vi "Mutate.RemoveOldInsertionPaletteItemsProject.vi"() -> ()   [LabVIEW 2013, in "VeriStand Steps Version Mutation.lvlib"]
uses:
  VeriStand Steps Version Mutation.lvlib
  <vilib>/xml/Load XML File.vi
  <vilib>/xml/Close Reference(Node).vi
  <vilib>/xml/Close Reference(NNMap).vi
  <vilib>/ni/Simple XML/_polymorphics/Create Tag - Child with Text.vi
  <vilib>/xml/NI_XML.lvlib
  <resource>/objmgr/DOMUserDefRef.rc
  <vilib>/ni/Simple XML/Simple XML.lvlib
panel:
  out "New Assembly Reference Include Strings":string[](array[string])=["NationalInstruments.TestStand.Interop.API, Version=1.2.3.4, Culture=neutral, PublicKeyToken=ad9244eb3b825cd8, processorArchitecture=MSIL", "NationalInstruments.TestStand.Interop.UI.AxControls, Version=1.2.3.4, Culture=neutral, PublicKeyToken=ad9244eb3b825cd8, processorArchitecture=MSIL", "NationalInstruments.TestStand.Interop.Utility, Version=5.6.7.8, Culture=neutral, processorArchitecture=x86"]
  out "New Assembly HintPath Properties":string[](array[string])=["..\\..\\..\\..\\..\\..\\..\\..\\..\\Program Files (x86)\\National Instruments\\TestStand 2013\\API\\DotNet\\Assemblies\\CurrentVersion\\NationalInstruments.TestStand.Interop.API.dll", "..\\..\\..\\..\\..\\..\\..\\..\\..\\Program Files (x86)\\National Instruments\\TestStand 2013\\API\\DotNet\\Assemblies\\CurrentVersion\\NationalInstruments.TestStand.Interop.UI.AxControls.dll", "..\\..\\..\\..\\..\\..\\..\\..\\..\\Program Files (x86)\\National Instruments\\TestStand 2013\\Bin\\NationalInstruments.TestStand.Utility.dll"]
  in  "New TS Version":dbl=2013.0 format="%#_6f"
  out "error out":errorcluster={"status"=TRUE, "code"=-2628, "source"="Invoke Node in NI_XML.lvlib:Load XML File.vi->Assembly Redirection VIs.lvlib:Redirect Assemblies in RemoveOldInsertionPaletteItems Project XML.vi"}
  in  "Path to New XML File":path=path "C:/Users/achurch/Documents/Source/XML Assembly Redirection Project/Examples XML Files/RemoveOldInsertionPaletteItems_mod.csproj" caption="Path to New RemoveOldInsertionPaletteItems project file"
  in  "New TS Utility Assembly Version":string="5.6.7.8"
  in  "New TS Interop Assembly Version":string="1.2.3.4"
  in  "XML file path":path=path "C:/Users/achurch/Documents/Source/XML Assembly Redirection Project/Examples XML Files/RemoveOldInsertionPaletteItems.csproj" caption="Path to Old RemoveOldInsertionPaletteItems project file"
  # "Arguments\n1: Old Project Path\n2: New Project Path\n3: New TS Version (2014)\n4: New TS Utility Version (2014.0.0.0)\n5: New TS Interop Version (2014.0.0.0)"
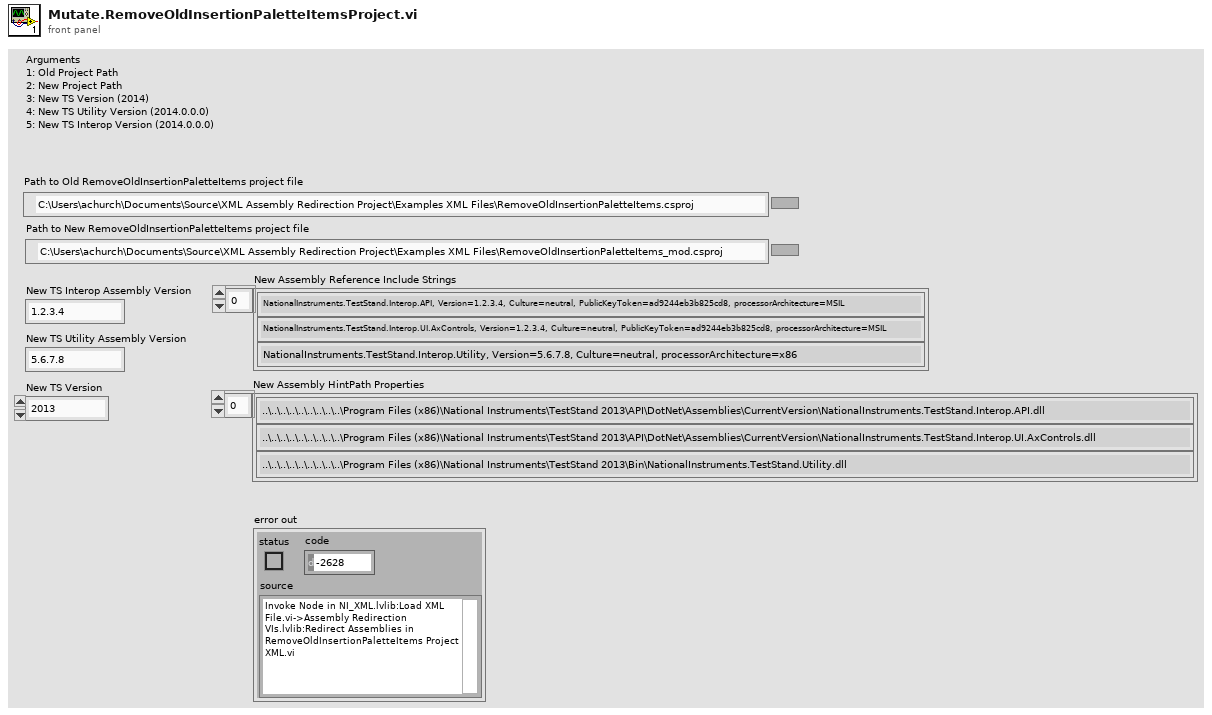
[diagram p1: front panel]
types:
  T1 = enum32{"invalid app kind", "Development System", "Run Time System", "Student Edition", "Embedded LabVIEW", "Evaluation", "Custom"}
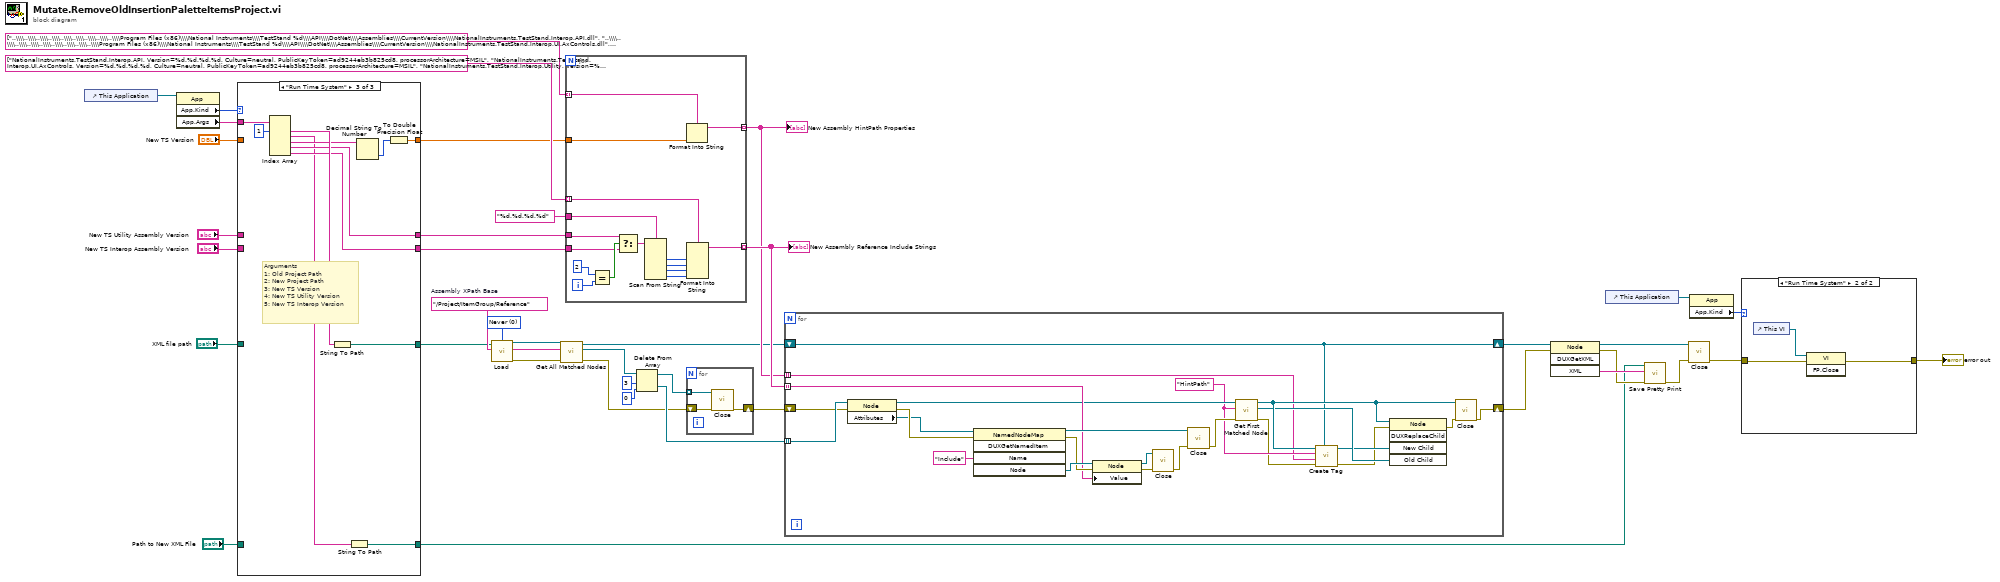
[diagram p0: block diagram]
diagram:
  w37 = "/Project/ItemGroup/Reference"  # Assembly XPath Base
  w40 = 0 items=["Never", "Always", "Auto"] ("validate on load (Auto)")
  n1 = control-ref of="This Application"() -> (w15:refnum<vi>)
  n2 = property class="App"(reference=w15) -> ("App.Kind"=w14:T1, "App.Args"=w13:string[])  [unwired: 1 in, 2 out]
  n3 = case shown="\"Run Time System\"" w14 {
    tunnel: "XML file path" -> [w44 w47 _]
    tunnel: "New TS Version" -> [w45 w50 _]
    tunnel: w13 -> [_ _ w61]
    tunnel: [w44 w47 w58] -> w12
    tunnel: [w42 w48 w56] -> w11
    tunnel: [w43 w49 w55] -> w10
    tunnel: [w45 w50 w53] -> w9
    tunnel: "New TS Utility Assembly Version" -> [w43 w49 _]
    tunnel: "New TS Interop Assembly Version" -> [w42 w48 _]
    tunnel: "Path to New XML File" -> [w41 w46 _]
    tunnel: [w41 w46 w51] -> w5
    frame Default {
    }
    frame "Development System" {
    }
    frame "Run Time System" {
      # "Arguments\n1: Old Project Path\n2: New Project Path\n3: New TS Version\n4: New TS Utility Version\n5: New TS Interop Version"
      n4 = Index Array(array=w61, index #1=1 ("index")) -> (element #1=w59:string, element #2=w52:string, element #3=w57:string, element #4=w55:string, element #5=w56:string)  [unwired: 4 in]
      n5 = String To Path(string=w59) -> (path=w58:path)
      n6 = String To Path(string=w52) -> (path=w51:path)
      n7 = Decimal String To Number(string=w57) -> (number=w54:i32)  [unwired: 2 in, 1 out]
      n8 = To Double Precision Float(number=w54) -> (double precision float=w53:dbl)
    }
  }
  n9 = call-poly <vilib>:"Load.vi"("path to XML document"=w12, "validate on load (Auto)"=w40) -> ("DOM document out"=w38:refnum<k20>, "error out"=w39:errorcluster)  [unwired: 11 in, 1 out]
  n10 = call <vilib>:"Get All Matched Nodes.vi"("error in (no error)"=w39, "XPath expression"=w37, "node in"=w38) -> ("error out"=w30:errorcluster, "node result array"=w35:refnum<k20>[], "node out"=w19:refnum<k20>)  [unwired: 6 in]
  n11 = for {
    tunnel: w10 -> [w73]
    tunnel: w11 -> [w74]
    tunnel: "%d.%d.%d.%d" ("format string") -> [w72]
    tunnel: string[] ["NationalInstruments.TestStand.Interop.API, Version=%d.%d.%d.%d, Culture=neutral, PublicKeyToken=ad9244eb3b825cd8, processorArchitecture=MSIL", "NationalInstruments.TestStand.Interop.UI.AxControls, Version=%d.%d.%d.%d, Culture=neutral, PublicKeyToken=ad9244eb3b825cd8, processorArchitecture=MSIL", "NationalInstruments.TestStand.Interop.Utility, Version=%d.%d.%d.%d, Culture=neutral, processorArchitecture=x86"] -> [w70] mode=indexing
    tunnel: [w65] -> w27 mode=indexing
    tunnel: string[] ["..\\\\..\\\\..\\\\..\\\\..\\\\..\\\\..\\\\..\\\\..\\\\Program Files (x86)\\\\National Instruments\\\\TestStand %d\\\\API\\\\DotNet\\\\Assemblies\\\\CurrentVersion\\\\NationalInstruments.TestStand.Interop.API.dll", "..\\\\..\\\\..\\\\..\\\\..\\\\..\\\\..\\\\..\\\\..\\\\Program Files (x86)\\\\National Instruments\\\\TestStand %d\\\\API\\\\DotNet\\\\Assemblies\\\\CurrentVersion\\\\NationalInstruments.TestStand.Interop.UI.AxControls.dll", "..\\\\..\\\\..\\\\..\\\\..\\\\..\\\\..\\\\..\\\\..\\\\Program Files (x86)\\\\National Instruments\\\\TestStand %d\\\\Bin\\\\NationalInstruments.TestStand.Utility.dll"] -> [w64] mode=indexing
    tunnel: w9 -> [w63]
    tunnel: [w62] -> w20 mode=indexing
    i -> [w77]
    n12 = Equal?(x=2, y=w77) -> (x = y?=w75:bool)
    n13 = Select(t=w73, s=w75, f=w74) -> (s? t:f=w71:string)
    n14 = Scan From String(format string=w72, input string=w71) -> (output 1=w69:i32, output 2=w68:i32, output 3=w67:i32, output 4=w66:i32)  [unwired: 6 in, 3 out]
    n15 = Format Into String(format string=w64, w63) -> (resulting string=w62:string)  [unwired: 2 in, 1 out]
    n16 = Format Into String(format string=w70, w69, w68, w67, w66) -> (resulting string=w65:string)  [unwired: 2 in, 1 out]
  }
  "New Assembly HintPath Properties" <- w20
  "New Assembly Reference Include Strings" <- w27
  n17 = Delete From Array(array=w35, length=3, index=0 ("length")) -> (deleted portion=w32:refnum<k20>[], array with subset deleted=w31:refnum<k20>[])
  n18 = for {
    tunnel: w31 -> [w80] mode=indexing
    shift-right: [w78] -> w29
    shift-left: w30 -> [w79]
    n19 = call-poly <vilib>:"Close.vi"("error in (no error)"=w79, "node"=w80) -> ("error out"=w78:errorcluster)  [unwired: 7 in]
  }
  n20 = for {
    tunnel: w32 -> [w101] mode=indexing
    shift-right: [w95] -> w26
    shift-left: w29 -> [w100]
    tunnel: w27 -> [w94] mode=indexing
    tunnel: w20 -> [w82] mode=indexing
    shift-right: [w81] -> w18
    shift-left: w19 -> [w81]
    w89 = "HintPath" ("XPath expression")
    n21 = property class="Node"(reference=w101, error in=w100) -> (reference out=w90:refnum<k20>, error out=w104:errorcluster, "Attributes"=w102:refnum<k20>)
    n22 = invoke class="NamedNodeMap" method="DUXGetNamedItem"(reference=w102, error in=w104, "Name"="Include") -> (reference out=w96:refnum<k20>, error out=w98:errorcluster, "Node"=w99:refnum<k20>)  [unwired: 2 in, 2 out]
    n23 = property class="Node"(reference=w99, error in=w98, "Value"=w94) -> (reference out=w97:refnum<k20>, error out=w93:errorcluster)
    n24 = call-poly <vilib>:"Close.vi"("error in (no error)"=w93, "node"=w97) -> ("error out"=w92:errorcluster)  [unwired: 7 in]
    n25 = call-poly <vilib>:"Close.vi"("error in (no error)"=w92, "named node map"=w96) -> ("error out"=w91:errorcluster)  [unwired: 7 in]
    n26 = call <vilib>:"Get First Matched Node.vi"("error in (no error)"=w91, "XPath expression"=w89, "node in"=w90) -> ("error out"=w88:errorcluster, "node result"=w86:refnum<k20>, "node out"=w87:refnum<k20>)  [unwired: 6 in]
    n27 = call-poly <vilib>:"Create Tag.vi"("DOM document reference"=w81, "error in (no error)"=w88, "Text Data"=w82, "Tag Name"=w89, "Parent Element reference"=w87) -> ("error out"=w84:errorcluster, "Child Element reference"=w85:refnum<k20>)  [unwired: 5 in]
    n28 = invoke class="Node" method="DUXReplaceChild"(reference=w87, error in=w84, "New Child"=w85, "Old Child"=w86) -> (error out=w83:errorcluster)  [unwired: 1 in, 4 out]
    n29 = call-poly <vilib>:"Close.vi"("error in (no error)"=w83, "node"=w87) -> ("error out"=w95:errorcluster)  [unwired: 7 in]
  }
  n30 = invoke class="Node" method="DUXGetXML"(reference=w18, error in=w26) -> (reference out=w22:refnum<k20>, error out=w24:errorcluster, "XML"=w25:string)  [unwired: 2 in, 1 out]
  n31 = control-ref of="This Application"() -> (w4:refnum<vi>)
  n32 = call <vilib>:"Save Pretty Print.vi"("error in (no error)"=w24, "Pretty XML String"=w25, "XML file path"=w5) -> ("error out"=w23:errorcluster)  [unwired: 7 in, 1 out]
  n33 = call-poly <vilib>:"Close.vi"("error in (no error)"=w23, "node"=w22) -> ("error out"=w2:errorcluster)  [unwired: 7 in]
  n34 = property class="App"(reference=w4) -> ("App.Kind"=w3:T1)  [unwired: 1 in, 2 out]
  n35 = case shown="\"Run Time System\"" w3 {
    tunnel: w2 -> [w105 w107]
    tunnel: [w105 w106] -> w1
    frame "Development System", Default {
    }
    frame "Run Time System" {
      n36 = control-ref of="This VI"() -> (w108:refnum<vi>)
      n37 = invoke class="VI" method="FP.Close"(reference=w108, error in=w107) -> (error out=w106:errorcluster)  [unwired: 1 in, 2 out]
    }
  }
  "error out" <- w1
